vi "Pulsed BPSK Modem.vi"() -> ()   [LabVIEW 2025]
uses:
  Shared/Pulse BPSK Configuration.ctl
  chdr/CHDR Header Layout.ctl
  <vilib>/Platform/TimedLoop/XDataNode/timing_clust.ctl
  <vilib>/Platform/TimedLoop/XDataNode/nitl_modes.ctl
  <vilib>/Platform/TimedLoop/XDataNode/wakeup.ctl
  <vilib>/DLsc/v1/FPGA/DLsc/Endpoint/Data Transfer Type.ctl
  <vilib>/DLsc/v1/FPGA/Aurora 64b66b/Aurora Port Identifier.ctl
  Shared/Public/Demodulator Control.ctl
  <vilib>/rvi/Emulation/niFpgaSctlEmulationGetInTimedLoop.vi
  <vilib>/rvi/Emulation/niFpgaEmulationReportErrorSimple.vi
  <vilib>/rvi/Emulation/niFpgaGetClockAttributes.vi
  <vilib>/rvi/Emulation/niFpgaCriticalErrorInLSC.vi
  <vilib>/eio/utilities/niEioResolveVilibRelativePath.vi
  <vilib>/rvi/interface/RandomDataEmulation/niFpgaRandomDataHandleErrors.vi
  <instrlib>/_niInstr/Basic Elements/v1/FPGA/Private/Count Up U32.vi
  <vilib>/rvi/Memory/Memory_Emulation/nirvimemoryFastEmulation.vi
  <vilib>/rvi/Memory/Memory_Emulation/nirvimemoryEmulation.vi
  <vilib>/rvi/Emulation/niFpgaEmulationIsFPGAContextNoSignature.vi
  <vilib>/rvi/DataTransferAndStorage/Container/Common/niFpgaContainerGetUniqueNameForEmu.vi
  <vilib>/rvi/Emulation/niFpgaProcessEmulError.vi
  <vilib>/rvi/errors/nirviReportUnexpectedCaseInternalError (U32).vi
  <vilib>/rvi/errors/niFpgaSetErrorForExecOnDevCompSimple.vi
  <vilib>/rvi/eio/common/nirviEmuReportErrorAndStop.vi
  <vilib>/rvi/FIFO/Fifo_Resource/nirvififoEmulationSetSize.vi
  <vilib>/rvi/FIFO/Fifo_Resource/nirviFifoEmulationQueueMgr.vi
  <instcachedir>/0/nirviFifoEmulationQueueMgr_E5CAEC123FF24DC58D834DCA3CDAA9B5.lvgen/nirviFifoEmulationQueueMgr_E5CAEC123FF24DC58D834DCA3CDAA9B5_015.vi
  <vilib>/Utility/error.llb/Clear Errors.vi
  <vilib>/rvi/FIFO/Fifo_Resource/nirvififoEmulationCreateLock.vi
  <vilib>/rvi/FIFO/Fifo_Resource/nirvififoEmulationObtainLock.vi
  <vilib>/rvi/FIFO/Fifo_Resource/nirvififoEmulationReleaseLock.vi
  <vilib>/rvi/occurrence/nirviWaitOnOccurrenceBase.vi
  <vilib>/rvi/errors/nirviReportUnexpectedCaseInternalError.vi
  <vilib>/rvi/DataTransferAndStorage/Container/Common/niFpgaContainerSetEmuInfo.vi
  <vilib>/DLsc/v1/FPGA/Aurora 64b66b/Create DX Advanced.vi
  <vilib>/DLsc/v1/FPGA/DLsc/Endpoint/Read Data Stream with Framing 256 Bits.vi
  <instrlib>/_niInstr/Data Formatting/v1/FPGA/Private/Convert/Boolean Array to U32 Array.vi
  <instrlib>/_niInstr/Basic Elements/v1/FPGA/Private/Count Up U64.vi
  <instrlib>/_niInstr/Data Formatting/v1/FPGA/Private/Convert/U32 array to Boolean Array.vi
  <vilib>/DLsc/v1/FPGA/DLsc/Endpoint/Write Data Stream with Framing 256 Bits.vi
  <vilib>/rvi/interface/RandomDataEmulation/nirviRandomDataMultiElementFPGAFIFO.vi
  <instcachedir>/0/nirviRandomDataMultiElementFPGAFIFO_BE2FF10D3D6E420AB0291A02835C249E.lvgen/nirviRandomDataMultiElementFPGAFIFO_BE2FF10D3D6E420AB0291A02835C249E_001.vi
  <instcachedir>/0/nirviRandomDataMultiElementFPGAFIFO_BE2FF10D3D6E420AB0291A02835C249E.lvgen/nirviRandomDataMultiElementFPGAFIFO_BE2FF10D3D6E420AB0291A02835C249E_005.vi
  <vilib>/rvi/FIFO/Fifo_Resource/nirvififoEmulationDetermineInputValidOut.vi
  <vilib>/Platform/TimedLoop/XDataNode/XDataNode.xnode
  <vilib>/rvi/DataTransferAndStorage/Container/XNode/niFpgaContainer.xnode
  <vilib>/rvi/interface/RandomDataEmulation/nirviRandomDataFpgaReadWriteTemplate.vi
  <vilib>/rvi/FIFO/Fifo_Resource/nirvififoEmulationRead.vi
  <vilib>/rvi/LocalResourceManager/LocalResourceManager.xnode
  <vilib>/rvi/interface/RandomDataEmulation/nirviRandomDataFpgaMultiElementTemplate.vi
  <vilib>/rvi/FIFO/Fifo_Resource/nirvififoEmulationWrite.vi
  Shared/BER/FPGA/BER/BER.lvclass
  <vilib>/Platform/TimedLoop/XDataNode/XDNodeRunTimeDep.lvlib
  <instrlib>/_niInstr/FIFO Register Bus/v1/FPGA/niInstr FIFO Register Bus v1 FPGA.lvclass
  <instrlib>/_niInstr/Basic Elements/v1/FPGA/niInstr Basic Elements v1 FPGA.lvlib
  Shared/Pulsed BPSK Modem Shared.lvlib
  Shared/Modems Shared.lvlib
  Shared/AWGN/FPGA/AWGN FPGA.lvlib
  Shared/FIR/FIR.lvlib
  <vilib>/DLsc/v1/FPGA/DLsc/Endpoint/Endpoint.lvclass
  <vilib>/DLsc/v1/FPGA/DLsc/Collection/Endpoint Collection.lvclass
  Shared/AGC/AGC v1 FPGA.lvlib
  <vilib>/DLsc/v1/FPGA/Aurora 64b66b/DLsc Aurora 64b66b v1 FPGA.lvlib
  chdr/CHDR Support.lvlib
  <instrlib>/_niInstr/Data Formatting/v1/FPGA/niInstr Data Formatting v1 FPGA.lvlib
panel:
  out "header count.1":u64
  out "error detection.1":T1
  out "last_timestamp.1":u64
  out "last_header.1":T2
  out "header count.0":u64
  out "error detection.0":T1
  out "last_timestamp.0":u64
  out "last_header.0":T2
  out "bit stream length.1":u32
  in  "update bit generation.1":bool
  in  "preamble write.1":cluster{"address":u32, "write":bool, "value":u8}
  out "current threshold.1":fxp<+/-,15,15>
  in  "preamble.1":i32=449838109 format="%.0x"
  in  "frequency tracking k1.1":fxp<+/-,25,-2>
  in  "frequency tracking k2.1":fxp<+/-,20,-6>
  out "demodulated bits overflow.1":bool
  out "constellation IQ overflow.1":bool
  in  "aurora debug.1":bool
  in  "demodulator control.1":i16
  in  "frame length.1":u16
  out "demodulated bits to BER overflow.1":bool
  in  "threshold precentile.1":fxp<+/-,10,1>=0.80078125 format="%#_10g"
  in  "match filter coefficients.1":T3
  out "aurora.1":bool
  out "current level.1":fxp<+,32,3>
  in  "AGC configurations.1":T4={"k1"=0.0, "k2"=0.0, "target level"=0.0, "level threshold"=0.20001220703125} {"level threshold" format="%#_16g"}
  out "AGC gain.1":fxp<+,19,3>
  in  "reset demodulator.1":bool
  out "pulse buffer underflow.1":bool
  in  "pulse configuration.1":T5={"On Symbol Count"=0, "Off Symbol Count"=7, "filter length"=15, "Preamble Count"=0}
  out "modulated data overflow.1":bool
  out "sink overflow.1":bool
  in  "clear debug.1":bool
  out "pulse control overflow.1":bool
  in  "reset modulator.1":bool
  in  "pulse shaping filter coefficients odd.1":T3
  in  "pulse shaping filter coefficients even.1":T3
  in  "enable modulator.1":bool
  in  "modulator configurations.1":T6 {"power scaling" format="%.16g"; "AWGN scaling" format="%.16g"}
  out "output fifo elements.1":u32
  in  "aurora frame length.1":u16
  in  "header parameters.1":T7
  in  "header parameters.0":T7
  in  "aurora frame length.0":u16
  out "output fifo elements.0":u32
  in  "reset demodulator.0":bool
  out "AGC gain.0":fxp<+,19,3>
  in  "AGC configurations.0":T4={"k1"=0.0, "k2"=0.0, "target level"=0.0, "level threshold"=0.20001220703125} {"level threshold" format="%#_16g"}
  in  "modulator configurations.0":T6 {"power scaling" format="%.16g"; "AWGN scaling" format="%.16g"}
  out "current level.0":fxp<+,32,3>
  out "aurora.0":bool
  in  "match filter coefficients.0":T3
  in  "threshold precentile.0":fxp<+/-,10,1>=0.80078125 format="%#_10g"
  in  "enable modulator.0":bool
  in  "pulse shaping filter coefficients even.0":T3
  in  "pulse shaping filter coefficients odd.0":T3
  out "demodulated bits to BER overflow.0":bool
  in  "preamble write.0":cluster{"address":u32, "write":bool, "value":u8}
  out "bit stream length.0":u32
  in  "update bit generation.0":bool
  in  "reset modulator.0":bool
  out "pulse buffer underflow.0":bool
  in  "pulse configuration.0":T5={"On Symbol Count"=0, "Off Symbol Count"=7, "filter length"=15, "Preamble Count"=0}
  out "modulated data overflow.0":bool
  out "sink overflow.0":bool
  in  "clear debug.0":bool
  out "pulse control overflow.0":bool
  in  "frame length.0":u16
  in  "demodulator control.0":i16
  in  "aurora debug.0":bool
  out "constellation IQ overflow.0":bool
  out "demodulated bits overflow.0":bool
  in  "frequency tracking k2.0":fxp<+/-,20,-6>
  in  "frequency tracking k1.0":fxp<+/-,25,-2>
  in  "preamble.0":i32=449838109 format="%.0x"
  out "current threshold.0":fxp<+/-,15,15>
  in  "fifo reg bus ctrl 0":u32
  out "fifo reg bus data 0":u64
  out "fifo reg bus status 0":u32
  # "Port 8 - Modulator/Demodulator"
  # "Port 9 - Modulator/Demodulator"
  # "Instruction Framework Host Interface. Please do not modify"
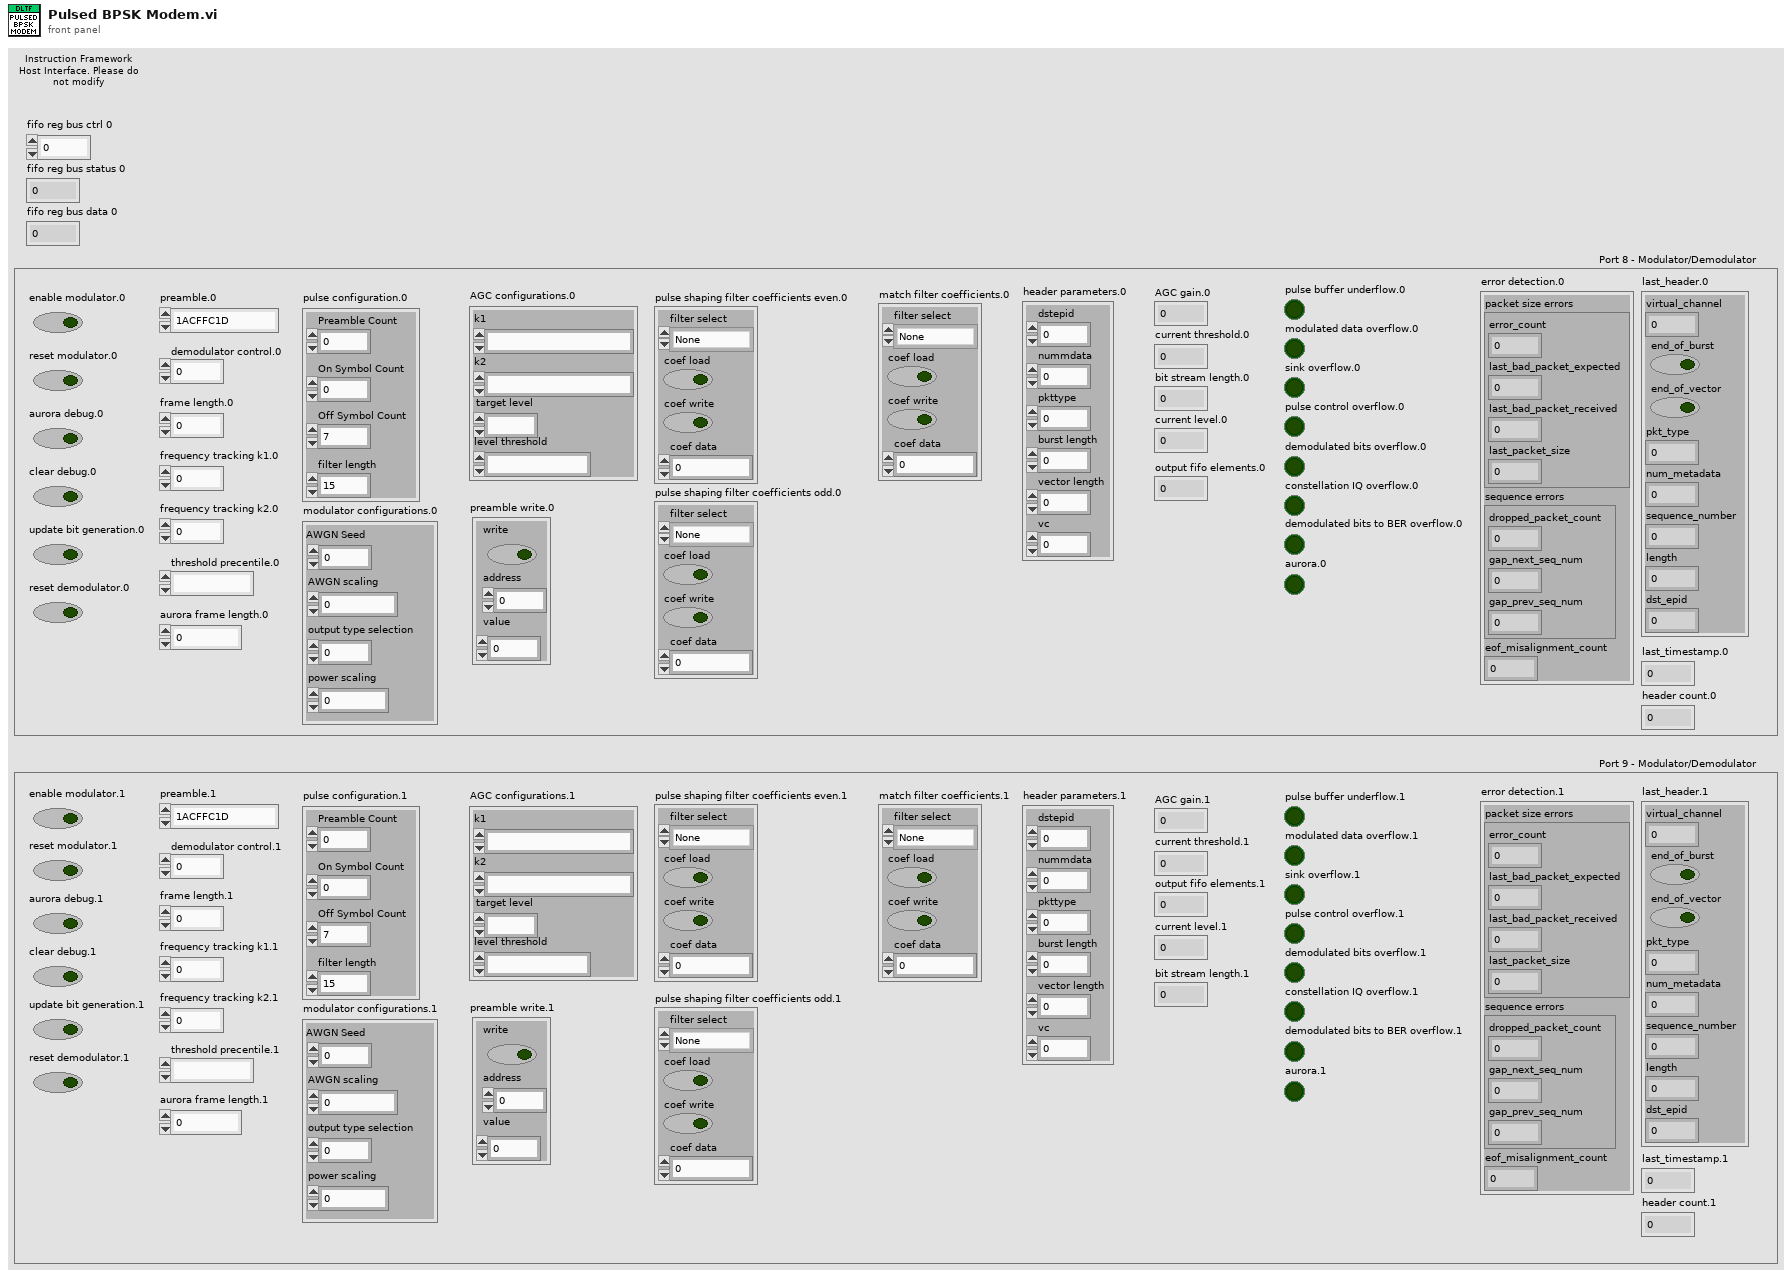
[diagram p1: front panel]
types:
  T1 = cluster{"packet size errors":cluster{"error_count":u64, "last_bad_packet_expected":u16, "last_bad_packet_received":u16, "last_packet_size":u16}, "sequence errors":cluster{"dropped_packet_count":u64, "gap_next_seq_num":u16, "gap_prev_seq_num":u16}, "eof_misalignment_count":u64}
  T2 = typedef "CHDR Support.lvlib/CHDR Header Layout.ctl" = cluster{"virtual_channel":fxp<+,6,6>, "end_of_burst":bool, "end_of_vector":bool, "pkt_type":fxp<+,3,3>, "num_metadata":fxp<+,5,5>, "sequence_number":u16, "length":u16, "dst_epid":u16}
  T3 = cluster{"filter select":enum8{"None", "I Inline", "I Cross", "Q Cross", "Q Inline"}, "coef load":bool, "coef write":bool, "coef data":fxp<+/-,18,1>}
  T4 = cluster{"k1":fxp<+,17,-4>, "k2":fxp<+,17,-8>, "target level":fxp<+,18,2>, "level threshold":fxp<+,18,4>}
  T5 = typedef "Modems Shared.lvlib/Pulse BPSK Configuration.ctl" = cluster{"On Symbol Count":u16, "Off Symbol Count":u16, "filter length":u16, "Preamble Count":u16}
  T6 = cluster{"AWGN Seed":fxp<+,25,25>, "AWGN scaling":fxp<+,16,0>, "output type selection":i16, "power scaling":fxp<+,16,0>}
  T7 = cluster{"dstepid":u16, "nummdata":fxp<+,5,5>, "pkttype":fxp<+,3,3>, "burst length":u16, "vector length":u16, "vc":fxp<+,6,6>}
  T8 = typedef "DLsc v1 FPGA.lvlib/Endpoint.lvclass/Data Transfer Type.ctl" = enum16{"u32 1spc", "u32 2spc", "u32 4spc", "u32 8spc", "u32 16spc", "u32 32spc"}
  T9 = typedef "DLsc Aurora 64b66b v1 FPGA.lvlib/Aurora Port Identifier.ctl" = enum16{"Port 0", "Port 1", "Port 2", "Port 3", "Port 4", "Port 5", "Port 6", "Port 7", "Port 8", "Port 9", "Port 10", "Port 11", "Ports 0-1", "Ports 2-3", "Ports 4-5", "Ports 6-7", "Ports 8-9", "Ports 10-11", "Ports 0-3", "Ports 4-7", "Ports 8-11"}
  T10 = typedef "XDNodeRunTimeDep.lvlib/timing_clust.ctl" = cluster{"Expected End [f-1]":u64, "Actual End [f-1]":u64, "Finished Late? [f-1]":bool, "Expected End [i-1]":u64, "Actual End [i-1]":u64, "Finished Late? [i-1]":bool, "Expected Start [i]":u64, "Actual Start [i]":u64, "Expected Start [f]":u64, "Actual Start [f]":u64, "Source Name":string, "Structure Name":string, "Period":i64, "Deadline":i64, "Offset":i64, "Start":i64, "Priority":i32, "Timeout":i32, "Mode":T11, "Wakeup Reason":T12, "Error":errorcluster, "Source Type":string, "Secondary Source Type":string, "Global End Time":u64, "Global Start Time":u64, "Frame Duration":u64, "Iteration Duration":u64, "Assigned CPU":i32, "I/O Scan Engine Mode":u32}
  T11 = typedef "XDNodeRunTimeDep.lvlib/nitl_modes.ctl" = enum32{"No Change", "Process missed periods, maintain original phase", "Discard missed periods, maintain original phase", "Process missed periods, ignore original phase", "Discard missed periods, ignore original phase"}
  T12 = typedef "XDNodeRunTimeDep.lvlib/wakeup.ctl" = enum32{"Normal", "Aborted", "Asynchronous wakeup", "Timing source error", "Timed loop error", "Timeout"}
  T13 = typedef "Pulsed BPSK Modem Shared.lvlib/Demodulator Control.ctl" = i16
  T14 = cluster{"dropped_packet_count":u64, "gap_next_seq_num":u16, "gap_prev_seq_num":u16}
  T15 = cluster{"error_count":u64, "last_bad_packet_expected":u16, "last_bad_packet_received":u16, "last_packet_size":u16}
  T16 = cluster{"magnitude":fxp<+,16,2>, "phase":fxp<+/-,16,1>, "output valid":bool}[]
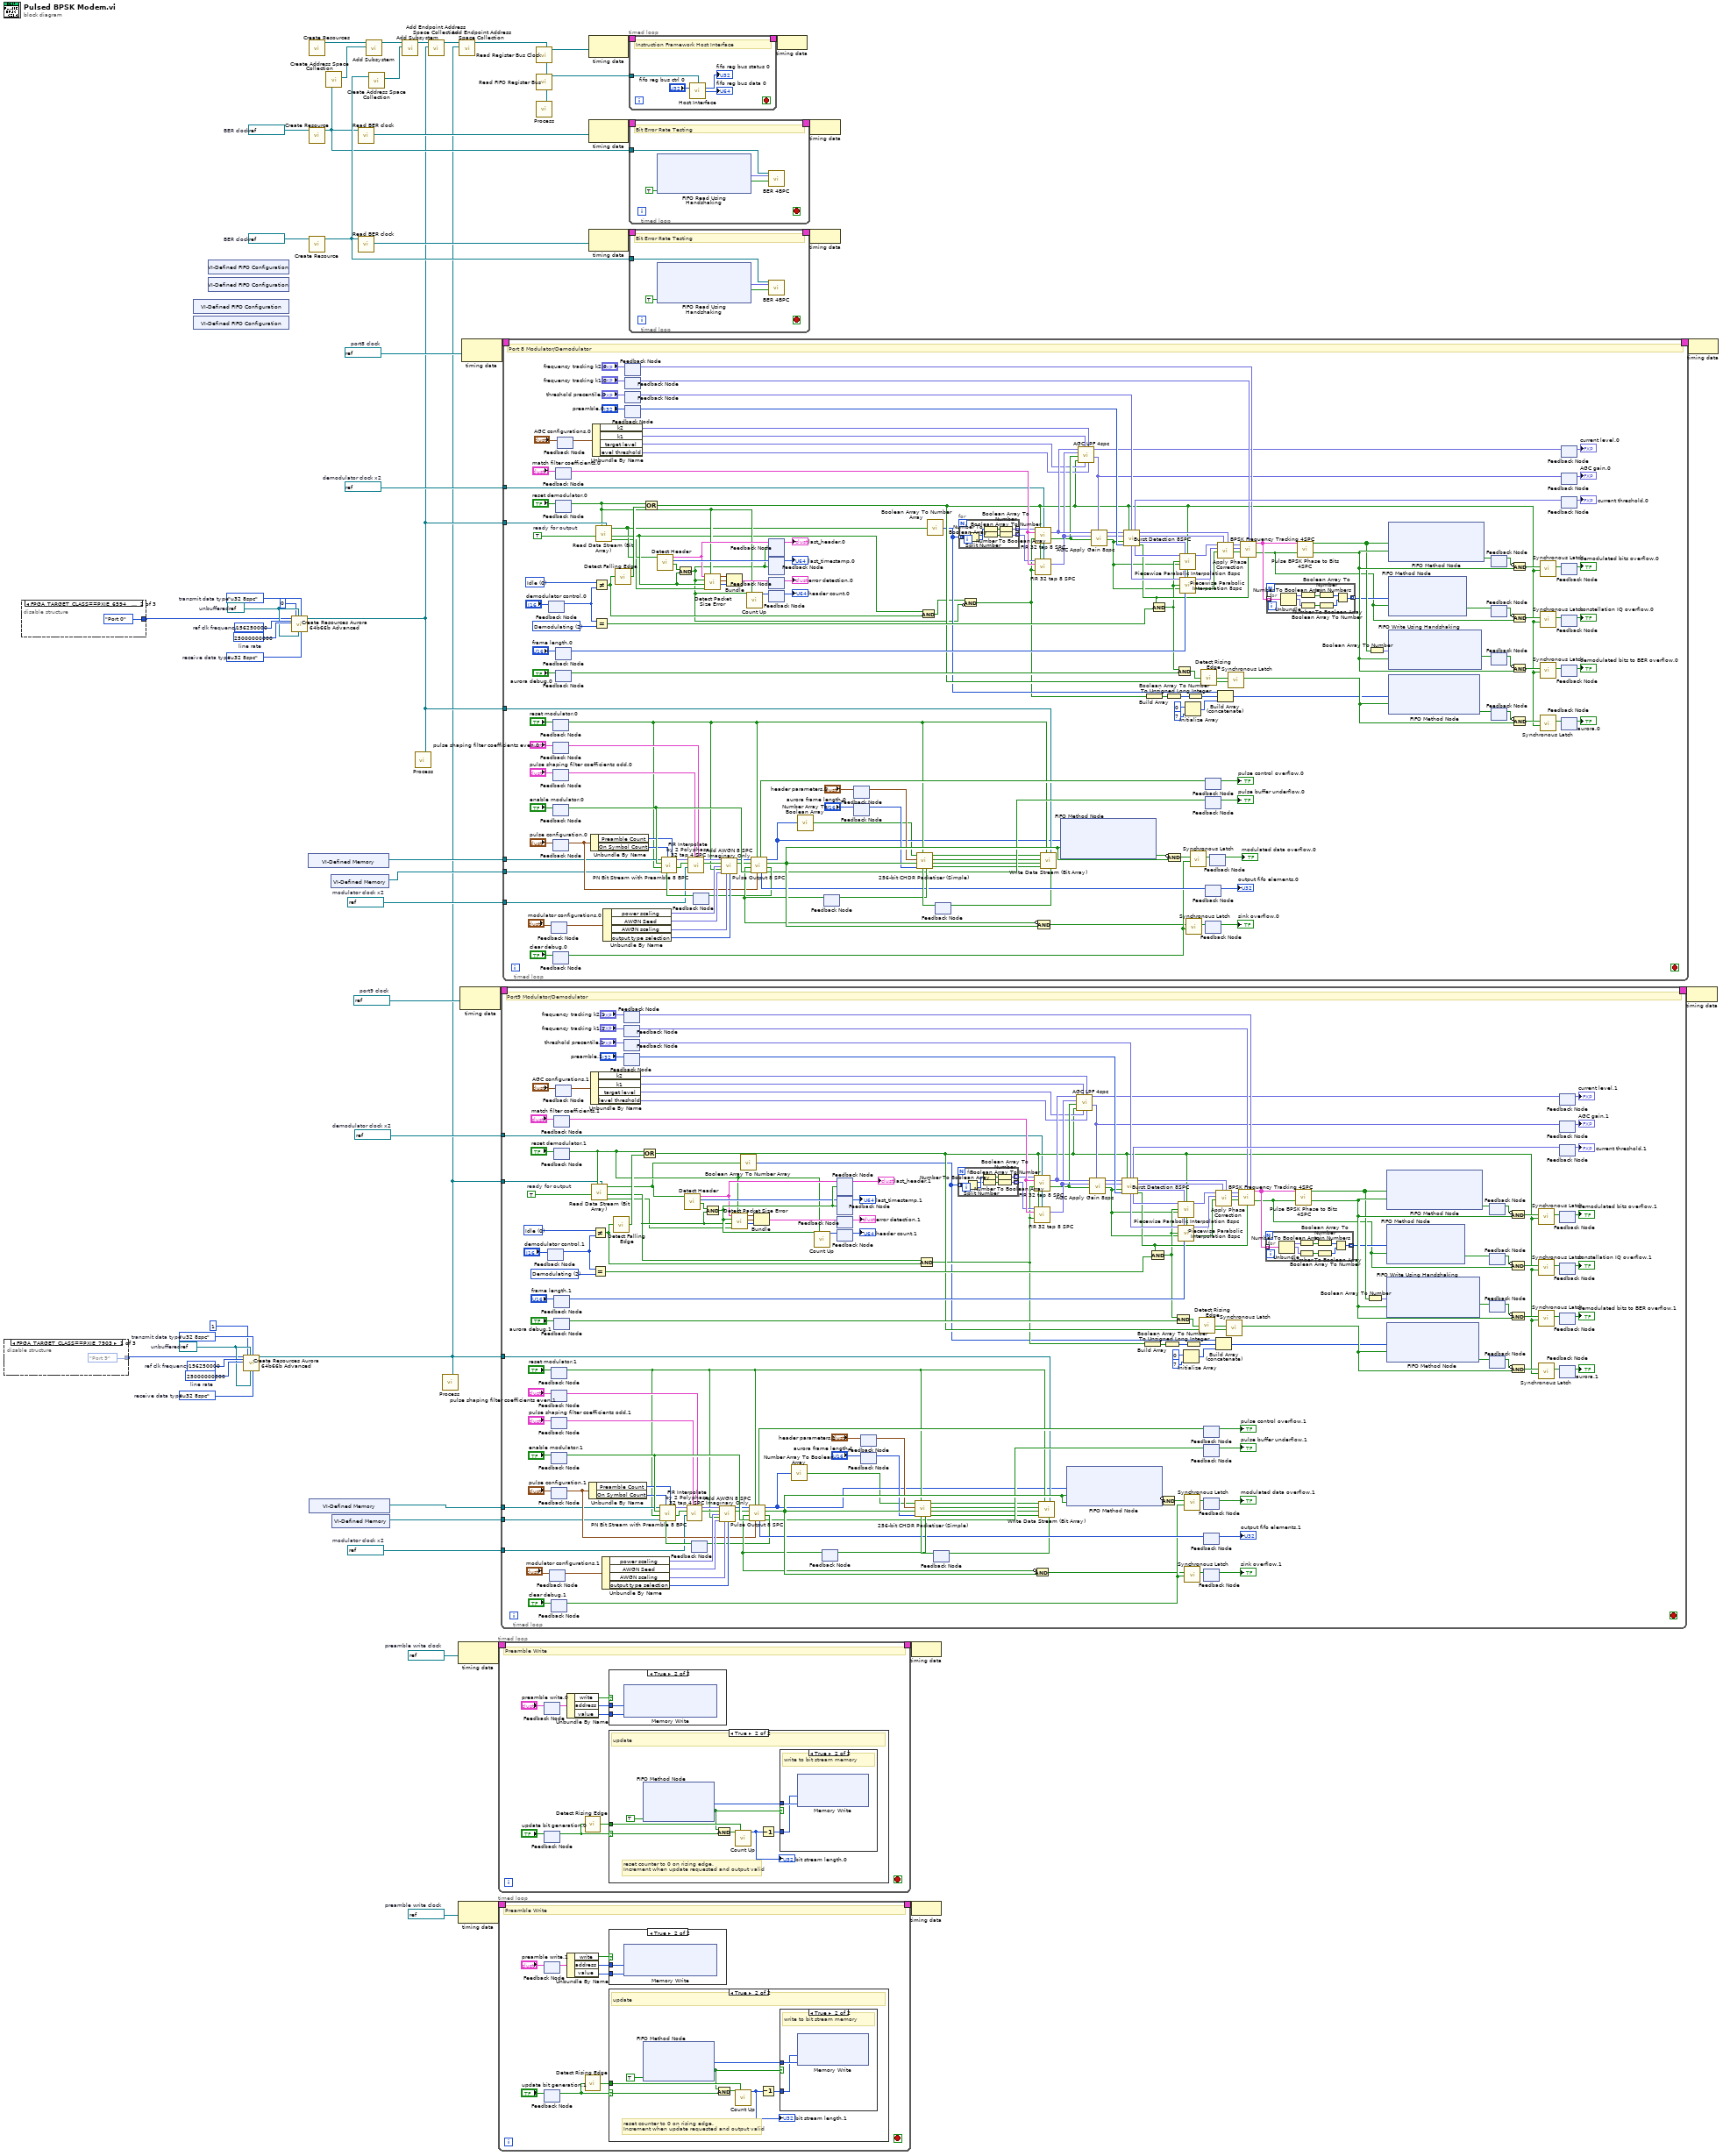
[diagram p0: block diagram]
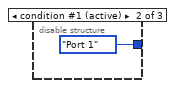
[diagram p2: hidden frame]
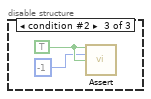
[diagram p3: hidden frame]
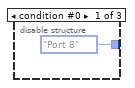
[diagram p4: hidden frame]
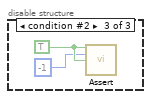
[diagram p5: hidden frame]
diagram:
  w4 = refnum<k21> refnum  # unbuffered
  w5 = Data_Transfer_Type."u32 8spc"  # transmit data type
  w7 = u64 25000000000  # line rate
  w6 = u64 156250000  # ref clk frequency
  w8 = Data_Transfer_Type."u32 8spc"  # receive data type
  w10 = refnum<k21> refnum  # unbuffered
  w11 = Data_Transfer_Type."u32 8spc"  # transmit data type
  w13 = u64 25000000000  # line rate
  w12 = u64 156250000  # ref clk frequency
  w14 = Data_Transfer_Type."u32 8spc"  # receive data type
  w26 = refnum<k21> "120MHz"  # BER clock
  w29 = refnum<k21> "120MHz"  # preamble write clock
  w32 = refnum<k21> "240MHz"  # modulator clock x2
  w33 = refnum<k21> "240MHz"  # demodulator clock x2
  w42 = refnum<k21> "240MHz"  # demodulator clock x2
  w43 = refnum<k21> "120MHz"  # port8 clock
  w37 = refnum<k21> "240MHz"  # modulator clock x2
  w47 = refnum<k21> "120MHz"  # BER clock
  w34 = refnum<k21> "120MHz"  # port9 clock
  w51 = refnum<k21> "120MHz"  # preamble write clock
  n1 = disable-structure shown="FPGA_TARGET_CLASS==PXIE_7903" {
    disable-tunnel: [Aurora_Port_Identifier."Port 9" ("aurora port identifier") Aurora_Port_Identifier."Port 1" ("aurora port identifier") _] -> w1
    frame condition #0 {
    }
    frame condition #1 (active) {
    }
    frame condition #2 {
      w61 = TRUE ("assert")
      n2 = call <instrlib>:"Assert.vi"("assert"=w61, "error code"=-1, "enable show error"=w61) -> ()  [unwired: 13 in]
    }
  }
  n3 = disable-structure shown="FPGA_TARGET_CLASS==PXIE_6594__KU15P_" {
    disable-tunnel: [Aurora_Port_Identifier."Port 8" ("aurora port identifier") Aurora_Port_Identifier."Port 0" ("aurora port identifier") _] -> w2
    frame condition #0 {
    }
    frame condition #1 (active) {
    }
    frame condition #2 {
      w65 = TRUE ("assert")
      n4 = call <instrlib>:"Assert.vi"("assert"=w65, "error code"=-1, "enable show error"=w65) -> ()  [unwired: 13 in]
    }
  }
  n5 = xnode "VI-Defined FIFO Configuration"() -> ()  [unwired: 1 out]
  n6 = xnode "VI-Defined FIFO Configuration"() -> ()  [unwired: 1 out]
  n7 = xnode "VI-Defined FIFO Configuration"() -> ()  [unwired: 1 out]
  n8 = xnode "VI-Defined FIFO Configuration"() -> ()  [unwired: 1 out]
  n9 = call-poly <vilib>:"Create Resources Aurora 64b66b Advanced.vi"("aurora port identifier"=w1, "ref clk frequency"=w12, "line rate"=w13, "instance (0)"=u8 1, "transmit buffer process clock"=w10, "receive buffer process clock"=w10, "transmit data type"=w11, "receive data type"=w14) -> ("endpoint"=w15:refnum<class "Endpoint.lvclass">)  [unwired: 11 in]
  n10 = call-poly <vilib>:"Create Resources Aurora 64b66b Advanced.vi"("aurora port identifier"=w2, "ref clk frequency"=w6, "line rate"=w7, "instance (0)"=u8 0, "transmit buffer process clock"=w4, "receive buffer process clock"=w4, "transmit data type"=w5, "receive data type"=w8) -> ("endpoint"=w16:refnum<class "Endpoint.lvclass">)  [unwired: 11 in]
  n11 = xnode "VI-Defined Memory"() -> ("Memory Out"=w39:refnum<k21>)
  n12 = call <vilib>:"Create Resources.vi"() -> ("endpoint collection"=w44:refnum<class "Endpoint Collection.lvclass">)  [unwired: 11 in]
  n13 = call "Create Resource.vi"("BER clock"=w26) -> ("BER"=w17:refnum<class "BER.lvclass">)  [unwired: 10 in]
  n14 = call "Create Resource.vi"("BER clock"=w47) -> ("BER"=w22:refnum<class "BER.lvclass">)  [unwired: 10 in]
  n15 = xnode "VI-Defined Memory"() -> ("Memory Out"=w28:refnum<k21>)
  n16 = call-dynamic "Create Address Space Collection.vi"("BER"=w17) -> ("address space collection"=w21:refnum<class "Address Space Collection.lvclass">)  [unwired: 9 in, 1 out]
  n17 = xnode "VI-Defined Memory"() -> ("Memory Out"=w38:refnum<k21>)
  n18 = xnode "VI-Defined Memory"() -> ("Memory Out"=w27:refnum<k21>)
  n19 = call "Read BER clock.vi"("BER"=w17) -> ("BER clock"=w23:refnum<k21>)  [unwired: 10 in]
  n20 = call "Read BER clock.vi"("BER"=w22) -> ("BER clock"=w48:refnum<k21>)  [unwired: 10 in]
  n21 = call <vilib>:"Add Subsystem.vi"("subsystems"=w21, "endpoint collection in"=w44) -> ("endpoint collection out"=w20:refnum<class "Endpoint Collection.lvclass">)  [unwired: 9 in]
  n22 = call-dynamic "Create Address Space Collection.vi"("BER"=w22) -> ("address space collection"=w18:refnum<class "Address Space Collection.lvclass">)  [unwired: 9 in, 1 out]
  n23 = call <vilib>:"Add Subsystem.vi"("subsystems"=w18, "endpoint collection in"=w20) -> ("endpoint collection out"=w19:refnum<class "Endpoint Collection.lvclass">)  [unwired: 9 in]
  n24 = call <vilib>:"Process.vi"("endpoint"=w16) -> ()  [unwired: 11 in]
  n25 = call <vilib>:"Add Endpoint Address Space Collection.vi"("endpoint"=w16, "endpoint collection in"=w19) -> ("endpoint collection out"=w41:refnum<class "Endpoint Collection.lvclass">)  [unwired: 9 in]
  n26 = call <vilib>:"Process.vi"("endpoint"=w15) -> ()  [unwired: 11 in]
  n27 = node-c288(w51) -> (w53:T10)
  n28 = node-c288(w29) -> (w31:T10)
  n29 = call <vilib>:"Add Endpoint Address Space Collection.vi"("endpoint"=w15, "endpoint collection in"=w41) -> ("endpoint collection out"=w40:refnum<class "Endpoint Collection.lvclass">)  [unwired: 9 in]
  n30 = node-c288(w34) -> (w36:T10)
  n31 = node-c288(w43) -> (w55:T10)
  n32 = timed-loop {
    timing: w53 -> [_]
    timing-out: [_] -> w52
    stop <- _ stop-if-true
    # "Preamble Write"
    n33 = feedback #1() -> (w66:cluster{"address":u32, "write":bool, "value":u8})  [unwired: 1 in]
    n34 = feedback-in #1("preamble write.0") -> ()
    n35 = feedback #2() -> (w72:bool)  [unwired: 1 in]
    n36 = feedback-in #2("update bit generation.0") -> ()
    n37 = Unbundle By Name(w66) -> ("write"=w69:bool, "address"=w70:u32, "value"=w68:u8)
    n38 = call <instrlib>:"Detect Rising Edge.vi"("signal"=w72) -> ("edge detected"=w71:bool)  [unwired: 14 in]
    n39 = case shown="True" w69 {
      tunnel: w70 -> [_ w75]
      tunnel: w68 -> [_ w74]
      frame False {
      }
      frame True {
        n40 = xnode ("Memory Write")("Address"=w75, "Data"=w74) -> ()  [unwired: 1 in, 1 out]
      }
    }
    n41 = case shown="True" w72 {
      selector: w72 -> [_ w80]
      tunnel: w71 -> [_ w83]
      frame False {
        # "Don't update"
      }
      frame True {
        # "reset counter to 0 on rising edge.\nIncrement when update requested and output valid"
        # "update"
        n42 = xnode ("FIFO Method Node")("Ready for Output"=TRUE) -> ("Element"=w82:u8, "Output Valid"=w78:bool)  [unwired: 1 in, 1 out]
        n43 = Compound Arithmetic op=AND(w78, w80) -> (w79:bool)
        n44 = call-poly <instrlib>:"Count Up.vi"("increment"=w79, "reset"=w83) -> ("count out"=w76:u32)  [unwired: 13 in]
        "bit stream length.0" <- w76
        n45 = Decrement(x=w76) -> (x-1=w77:u32)
        n46 = case shown="True" w78 {
          tunnel: w77 -> [_ w84]
          tunnel: w82 -> [_ w85]
          frame False {
            # "nothing to write"
          }
          frame True {
            # "write to bit stream memory"
            n47 = xnode ("Memory Write")("Address"=w84, "Data"=w85) -> ()  [unwired: 1 in, 1 out]
          }
        }
      }
    }
  }
  n48 = timed-loop {
    timing: w31 -> [_]
    timing-out: [_] -> w30
    stop <- _ stop-if-true
    # "Preamble Write"
    n49 = feedback #3() -> (w88:cluster{"address":u32, "write":bool, "value":u8})  [unwired: 1 in]
    n50 = feedback-in #3("preamble write.1") -> ()
    n51 = feedback #4() -> (w94:bool)  [unwired: 1 in]
    n52 = feedback-in #4("update bit generation.1") -> ()
    n53 = Unbundle By Name(w88) -> ("write"=w91:bool, "address"=w92:u32, "value"=w90:u8)
    n54 = call <instrlib>:"Detect Rising Edge.vi"("signal"=w94) -> ("edge detected"=w93:bool)  [unwired: 14 in]
    n55 = case shown="True" w91 {
      tunnel: w92 -> [_ w97]
      tunnel: w90 -> [_ w96]
      frame False {
      }
      frame True {
        n56 = xnode ("Memory Write")("Address"=w97, "Data"=w96) -> ()  [unwired: 1 in, 1 out]
      }
    }
    n57 = case shown="True" w94 {
      selector: w94 -> [_ w102]
      tunnel: w93 -> [_ w105]
      frame False {
        # "Don't update"
      }
      frame True {
        # "reset counter to 0 on rising edge.\nIncrement when update requested and output valid"
        # "update"
        n58 = xnode ("FIFO Method Node")("Ready for Output"=TRUE) -> ("Element"=w104:u8, "Output Valid"=w100:bool)  [unwired: 1 in, 1 out]
        n59 = Compound Arithmetic op=AND(w100, w102) -> (w101:bool)
        n60 = call-poly <instrlib>:"Count Up.vi"("increment"=w101, "reset"=w105) -> ("count out"=w98:u32)  [unwired: 13 in]
        "bit stream length.1" <- w98
        n61 = Decrement(x=w98) -> (x-1=w99:u32)
        n62 = case shown="True" w100 {
          tunnel: w99 -> [_ w106]
          tunnel: w104 -> [_ w107]
          frame False {
            # "nothing to write"
          }
          frame True {
            # "write to bit stream memory"
            n63 = xnode ("Memory Write")("Address"=w106, "Data"=w107) -> ()  [unwired: 1 in, 1 out]
          }
        }
      }
    }
  }
  n64 = timed-loop {
    timing: w36 -> [_]
    timing-out: [_] -> w35
    tunnel: w33 -> [w191]
    tunnel: w28 -> [w141]
    tunnel: w27 -> [w140]
    tunnel: w32 -> [w139]
    tunnel: w15 -> [w120]
    tunnel: w15 -> [w115]
    stop <- _ stop-if-true
    w138 = TRUE  # ready for output
    w268 = T13 2 items=["Idle", "Initial Threshold Detection", "Demodulating"] ("demodulation control")
    w271 = T13 0 items=["Idle", "Initial Threshold Detection", "Demodulating"] ("demodulation control")
    # "Port9 Modulator/Demodulator"
    n65 = feedback #5() -> (w269:i16)  [unwired: 1 in]
    n66 = feedback-in #5("demodulator control.1") -> ()
    n67 = feedback #6() -> (w175:T6)  [unwired: 1 in]
    n68 = feedback-in #6("modulator configurations.1") -> ()
    n69 = feedback #7() -> (w119:bool)  [unwired: 1 in]
    n70 = feedback-in #7("reset modulator.1") -> ()
    n71 = feedback #8() -> (w167:T3)  [unwired: 1 in]
    n72 = feedback-in #8("pulse shaping filter coefficients even.1") -> ()
    n73 = feedback #9() -> (w166:T3)  [unwired: 1 in]
    n74 = feedback-in #9("pulse shaping filter coefficients odd.1") -> ()
    n75 = feedback #10() -> (w180:bool)  [unwired: 1 in]
    n76 = feedback-in #10("enable modulator.1") -> ()
    n77 = feedback #11() -> (w142:T5)  [unwired: 1 in]
    n78 = feedback-in #11("pulse configuration.1") -> ()
    n79 = feedback #12() -> (w158:bool)  [unwired: 1 in]
    n80 = feedback-in #12("clear debug.1") -> ()
    n81 = feedback #13() -> (w254:T3)  [unwired: 1 in]
    n82 = feedback-in #13("match filter coefficients.1") -> ()
    n83 = feedback #14() -> (w123:bool)  [unwired: 1 in]
    n84 = feedback-in #14("reset demodulator.1") -> ()
    n85 = feedback #15() -> (w238:u16)  [unwired: 1 in]
    n86 = feedback-in #15("frame length.1") -> ()
    n87 = feedback #16() -> (w211:bool)  [unwired: 1 in]
    n88 = feedback-in #16("aurora debug.1") -> ()
    n89 = feedback-in #17("AGC configurations.1") -> ()
    n90 = feedback #17() -> (w200:T4)  [unwired: 1 in]
    n91 = Unbundle By Name(w142) -> ("Preamble Count"=w147:u16, "On Symbol Count"=w155:u16)
    n92 = Unbundle By Name(w200) -> ("k2"=w198:fxp<+,17,-8>, "k1"=w199:fxp<+,17,-4>, "target level"=w197:fxp<+,18,2>, "level threshold"=w196:fxp<+,18,4>)
    n93 = call-poly <vilib>:"Read Data Stream (Bit Array).vi"("endpoint"=w115, "reset"=w123, "ready for output"=w138) -> ("end of frame"=w114:bool, "output valid"=w124:bool, "data"=w122:bool[])  [unwired: 5 in, 1 out]
    n94 = Not Equal?(x=w271, y=w269) -> (x != y?=w262:bool)
    n95 = Equal?(x=w269, y=w268) -> (x = y?=w242:bool)
    n96 = Unbundle By Name(w175) -> ("power scaling"=w176:fxp<+,16,0>, "AWGN Seed"=w177:fxp<+,25,25>, "AWGN scaling"=w178:fxp<+,16,0>, "output type selection"=w179:i16)
    n97 = call <instrlib>:"Detect Falling Edge.vi"("signal"=w262) -> ("edge detected"=w263:bool)  [unwired: 14 in]
    n98 = feedback #18() -> (w244:fxp<+/-,20,-6>)  [unwired: 1 in]
    n99 = feedback-in #18("frequency tracking k2.1") -> ()
    n100 = feedback #19() -> (w245:fxp<+/-,25,-2>)  [unwired: 1 in]
    n101 = feedback-in #19("frequency tracking k1.1") -> ()
    n102 = feedback #20() -> (w247:fxp<+/-,10,1>)  [unwired: 1 in]
    n103 = feedback-in #20("threshold precentile.1") -> ()
    n104 = feedback #21() -> (w248:i32)  [unwired: 1 in]
    n105 = feedback-in #21("preamble.1") -> ()
    n106 = Compound Arithmetic op=OR(w123, w263) -> (w192:bool)
    n107 = call "Detect Header.vi"("input data"=w122) -> ("header detected"=w134:bool, "timestamp"=w136:u64, "chdr_header"=w135:T2)  [unwired: 8 in]
    n108 = feedback #22() -> (w164:bool)  [unwired: 1 in]
    n109 = call "PN Bit Stream with Preamble 8 BPC.vi"("preamble count"=w147, "ready for output"=w164, "on symbol count"=w155, "bit stream memory"=w140, "reset modulator"=w119, "start modulator"=w180, "preamble memory"=w141) -> ("output valid"=w169:bool, "data"=w168:fxp<+/-,16,1>[])  [unwired: 3 in]
    n110 = call "FIR Interpolate by 2 Polyphase 32 tap 4 SPC.vi"("filter coefficients even"=w167, "filter coefficients odd"=w166, "clock x2"=w139, "input valid"=w169, "data"=w168) -> ("output valid"=w171:bool, "data out"=w170:fxp<+/-,16,2>[])  [unwired: 5 in]
    n111 = Compound Arithmetic op=AND(w134, w124) -> (w137:bool)
    n112 = call "Add AWGN 8 SPC Imaginary Only.vi"("imaginary"=w170, "input valid"=w171, "power scaling"=w176, "reset"=w119, "seed"=w177, "scaling factor"=w178, "Output Type Selection"=w179) -> ("output with noise"=w162:u32[], "output valid"=w163:bool)  [unwired: 7 in]
    n113 = call "Detect Packet Size Error.vi"("reset_pse"=w123, "end of frame"=w114, "input valid"=w124, "packet_header"=w137, "chdr_header"=w135) -> ("eof_misalignment_count"=w129:u64, "sequence errors"=w128:T14, "packet size errors"=w127:T15)  [unwired: 4 in]
    n114 = call-poly <instrlib>:"Boolean Array To Number Array.vi"("data in"=w122) -> ("data out"=w121:u32[])  [unwired: 14 in]
    n115 = Bundle("packet size errors"=w127, "sequence errors"=w128, "eof_misalignment_count"=w129) -> (w131:T1)  [unwired: 1 in]
    n116 = call-poly <instrlib>:"Count Up.vi"("increment"=w137, "reset"=w123) -> ("count out"=w130:u64)  [unwired: 13 in]
    n117 = feedback #23() -> (w157:bool)  [unwired: 1 in]
    n118 = call "Pulse Output 8 SPC.vi"("Pulse Configuration"=w142, "reset"=w119, "enable"=w180, "ready for output"=w157, "input valid"=w163, "8 spc imaginary"=w162) -> ("Pulse Buffer Underflow"=w143:bool, "Ready for Input"=w144:bool, "output valid"=w187:bool, "IQ data out"=w113:u32[], "Number of Elements to Read"=w181:u32, "pulse buffer overflow"=w172:bool)
    n119 = feedback-in #22(w144) -> ()
    n120 = call-poly <instrlib>:"Number Array To Boolean Array.vi"("data in"=w113) -> ("data out"=w112:bool[])  [unwired: 14 in]
    n121 = feedback #24() -> (→"last_header.1":T2)  [unwired: 1 in]
    n122 = feedback-in #24(w135, w137) -> ()
    n123 = feedback #25() -> (→"last_timestamp.1":u64)  [unwired: 1 in]
    n124 = feedback-in #25(w136, w137) -> ()
    n125 = feedback #26() -> (→"error detection.1":T1)  [unwired: 1 in]
    n126 = feedback-in #26(w131) -> ()
    n127 = feedback #27() -> (→"header count.1":u64)  [unwired: 1 in]
    n128 = feedback-in #27(w130) -> ()
    n129 = feedback #28() -> (w184:T7)  [unwired: 1 in]
    n130 = feedback-in #28("header parameters.1") -> ()
    n131 = feedback #29() -> (w186:u16)  [unwired: 1 in]
    n132 = feedback-in #29("aurora frame length.1") -> ()
    n133 = Compound Arithmetic op=AND(w124, w262) -> (w190:bool)
    n134 = feedback #30() -> (w189:bool)  [unwired: 1 in]
    n135 = call "256-bit CHDR Packetizer (Simple).vi"("ready for output"=w189, "reset"=w119, "aurora frame length"=w186, "input valid"=w187, "header parameters"=w184, "data"=w112) -> ("tlast"=w110:bool, "output valid"=w116:bool, "tkeep"=w111:bool[], "data out"=w118:bool[], "ready for input"=w188:bool)  [unwired: 1 in]
    n136 = feedback-in #23(w188) -> ()
    n137 = for {
      tunnel: w121 -> [w286] mode=indexing
      tunnel: [w285] -> w253 mode=indexing
      tunnel: [w284] -> w252 mode=indexing
      n138 = Split Number(x=w286) -> (hi(x)=w289:u16, lo(x)=w290:u16)
      n139 = Number To Boolean Array(number=w290) -> (Boolean array=w288:bool[])
      n140 = Number To Boolean Array(number=w289) -> (Boolean array=w287:bool[])
      n141 = Boolean Array To Number(Boolean array=w288) -> (number=w285:fxp<+/-,16,1>)
      n142 = Boolean Array To Number(Boolean array=w287) -> (number=w284:fxp<+/-,16,1>)
    }
    n143 = call "FIR 32 tap 8 SPC.vi"("data in"=w253, "reset"=w192, "clock x2"=w191, "filter coefficients"=w254, "input valid"=w190) -> ("data out 16.1"=w209:fxp<+/-,16,1>[], "output valid"=w207:bool)  [unwired: 8 in, 1 out]
    n144 = call "FIR 32 tap 8 SPC.vi"("data in"=w252, "reset"=w192, "clock x2"=w191, "filter coefficients"=w254, "input valid"=w190) -> ("data out 16.1"=w208:fxp<+/-,16,1>[])  [unwired: 8 in, 2 out]
    n145 = Compound Arithmetic op=AND(invert w157, w187) -> (w153:bool)
    n146 = call-poly <vilib>:"Write Data Stream (Bit Array).vi"("endpoint"=w120, "reset"=w119, "end of frame"=w110, "input valid"=w116, "byte enable"=w111, "data"=w118) -> ("ready for input"=w117:bool)  [unwired: 5 in]
    n147 = feedback-in #30(w117) -> ()
    n148 = xnode ("FIFO Method Node")("Element"=w113, "Input Valid"=w187) -> ("Ready for Input"=w148:bool)  [unwired: 1 in, 1 out]
    n149 = call "AGC LPF 4spc.vi"("level threshold"=w196, "k 2"=w198, "level"=w197, "k 1"=w199, "reset"=w192, "input valid"=w207, "din img"=w208, "din real"=w209) -> ("AGC gain"=w194:fxp<+,19,3>, "current level"=w203:fxp<+,32,3>)  [unwired: 1 in, 1 out]
    n150 = call "AGC Apply Gain 8spc.vi"("AGC gain"=w194, "input valid"=w207, "din img"=w208, "din real"=w209) -> ("output valid"=w204:bool, "dout img"=w205:fxp<+/-,16,1>[], "dout real"=w206:fxp<+/-,16,1>[])  [unwired: 5 in]
    n151 = call "Burst Detection 8SPC.vi"("x real"=w206, "reset"=w192, "threshold precentile"=w247, "x img"=w205, "input valid"=w204, "preamble"=w248) -> ("Current Threshold"=w246:fxp<+/-,15,15>, "phase correction cos"=w237:fxp<+/-,16,2>, "phase correction sin"=w236:fxp<+/-,16,2>, "timing"=w243:fxp<+,13,0>, "img to interpolator"=w228:fxp<+/-,16,1>[], "real to interpolator"=w229:fxp<+/-,16,1>[], "preamble detected"=w226:bool)  [unwired: 2 in, 1 out]
    n152 = Build Array(w190) -> (w213:bool[])
    n153 = Compound Arithmetic op=AND(w226, w242) -> (w212:bool)
    n154 = Compound Arithmetic op=AND(invert w148, w187) -> (w149:bool)
    n155 = Boolean Array To Number(Boolean array=w213) -> (number=w219:u8)
    n156 = Compound Arithmetic op=AND(w212, w211) -> (w210:bool)
    n157 = call "Piecewise Parabolic Interpolation 8spc.vi"("x[n]"=w229, "u[k]"=w243, "reset"=w192, "preamble found"=w212, "input valid"=w204, "frame length"=w238) -> ("y[n]"=w234:fxp<+/-,16,2>[])  [unwired: 8 in, 1 out]
    n158 = call "Piecewise Parabolic Interpolation 8spc.vi"("x[n]"=w228, "u[k]"=w243, "reset"=w192, "preamble found"=w212, "input valid"=w204, "frame length"=w238) -> ("y[n]"=w233:fxp<+/-,16,2>[], "output valid"=w230:bool)  [unwired: 8 in]
    n159 = Initialize Array(u32 0 ("element"), 7 ("dimension size")) -> (w217:u32[])
    n160 = call <instrlib>:"Synchronous Latch.vi"("clear"=w158, "set"=w149) -> ("out"=w150:bool)  [unwired: 9 in]
    n161 = call <instrlib>:"Synchronous Latch.vi"("clear"=w158, "set"=w153) -> ("out"=w152:bool)  [unwired: 9 in]
    n162 = To Unsigned Long Integer(number=w219) -> (unsigned 32bit integer=w218:u32)
    n163 = call <instrlib>:"Detect Rising Edge.vi"("signal"=w210) -> ("edge detected"=w227:bool)  [unwired: 14 in]
    n164 = feedback #31() -> (→"pulse control overflow.1":bool)  [unwired: 1 in]
    n165 = feedback-in #31(w172) -> ()
    n166 = feedback #32() -> (→"pulse buffer underflow.1":bool)  [unwired: 1 in]
    n167 = feedback-in #32(w143) -> ()
    n168 = feedback #33() -> (→"modulated data overflow.1":bool)  [unwired: 1 in]
    n169 = feedback-in #33(w150) -> ()
    n170 = feedback #34() -> (→"output fifo elements.1":u32)  [unwired: 1 in]
    n171 = feedback-in #34(w181) -> ()
    n172 = feedback #35() -> (→"sink overflow.1":bool)  [unwired: 1 in]
    n173 = feedback-in #35(w152) -> ()
    n174 = call "Apply Phase Correction.vi"("phase correction cos"=w237, "phase correction sin"=w236, "input valid"=w230, "input img"=w233, "input real"=w234) -> ("output valid"=w249:bool, "output img"=w250:fxp<+/-,16,2>[], "output real"=w251:fxp<+/-,16,2>[])  [unwired: 4 in]
    n175 = Build Array (concatenate)(w121, w218, w217) -> (w214:u32[])
    n176 = call <instrlib>:"Synchronous Latch.vi"("clear"=w192, "set"=w227) -> ("out"=w220:bool)  [unwired: 9 in]
    n177 = call "BPSK Frequency Tracking 4SPC.vi"("I data in"=w251, "k1"=w245, "k2"=w244, "Q data in"=w250, "input valid"=w249, "reset"=w226) -> ("polar output"=w235:T16, "output valid"=w231:bool)  [unwired: 7 in, 1 out]
    n178 = for {
      tunnel: [w294] -> w232 mode=indexing
      tunnel: w235 -> [w293] mode=indexing
      n179 = Unbundle(w293) -> ("magnitude"=w292:fxp<+,16,2>, "phase"=w291:fxp<+/-,16,1>)  [unwired: 1 out]
      n180 = Number To Boolean Array(number=w292) -> (Boolean array=w298:bool[])
      n181 = Number To Boolean Array(number=w291) -> (Boolean array=w297:bool[])
      n182 = Boolean Array To Number(Boolean array=w298) -> (number=w296:u16)
      n183 = Boolean Array To Number(Boolean array=w297) -> (number=w295:u16)
      n184 = Join Numbers(hi=w296, lo=w295) -> ((hi.lo)=w294:u32)
    }
    n185 = call "Pulse BPSK Phase to Bits 4SPC.vi"("polar output"=w235, "input valid"=w231) -> ("bit"=w239:bool[], "output valid"=w241:bool)  [unwired: 12 in]
    n186 = Boolean Array To Number(Boolean array=w239) -> (number=w240:fxp<+,4,4>)
    n187 = xnode ("FIFO Method Node")("Element"=w239, "Input Valid"=w241) -> ("Ready for Input"=w267:bool)  [unwired: 1 in, 1 out]
    n188 = xnode ("FIFO Method Node")("Element"=w232, "Input Valid"=w231) -> ("Ready for Input"=w265:bool)  [unwired: 1 in, 1 out]
    n189 = xnode ("FIFO Write Using Handshaking")("Element"=w240, "Input Valid"=w241) -> ("Ready for Input"=w257:bool)  [unwired: 1 in, 1 out]
    n190 = xnode ("FIFO Method Node")("Element"=w214, "Input Valid"=w220) -> ("Ready for Input"=w225:bool)  [unwired: 1 in, 1 out]
    n191 = feedback #36() -> (w266:bool)  [unwired: 1 in]
    n192 = feedback-in #36(w267) -> ()
    n193 = feedback #37() -> (w264:bool)  [unwired: 1 in]
    n194 = feedback-in #37(w265) -> ()
    n195 = feedback #38() -> (w258:bool)  [unwired: 1 in]
    n196 = feedback-in #38(w257) -> ()
    n197 = feedback #39() -> (w221:bool)  [unwired: 1 in]
    n198 = feedback-in #39(w225) -> ()
    n199 = Compound Arithmetic op=AND(invert w266, w241) -> (w279:bool)
    n200 = Compound Arithmetic op=AND(invert w264, w231) -> (w276:bool)
    n201 = Compound Arithmetic op=AND(invert w258, w241) -> (w259:bool)
    n202 = Compound Arithmetic op=AND(invert w221, w220) -> (w222:bool)
    n203 = call <instrlib>:"Synchronous Latch.vi"("clear"=w192, "set"=w279) -> ("out"=w278:bool)  [unwired: 9 in]
    n204 = call <instrlib>:"Synchronous Latch.vi"("clear"=w192, "set"=w276) -> ("out"=w275:bool)  [unwired: 9 in]
    n205 = call <instrlib>:"Synchronous Latch.vi"("clear"=w192, "set"=w259) -> ("out"=w260:bool)  [unwired: 9 in]
    n206 = call <instrlib>:"Synchronous Latch.vi"("clear"=w192, "set"=w222) -> ("out"=w223:bool)  [unwired: 9 in]
    n207 = feedback #40() -> (→"current level.1":fxp<+,32,3>)  [unwired: 1 in]
    n208 = feedback-in #40(w203) -> ()
    n209 = feedback #41() -> (→"AGC gain.1":fxp<+,19,3>)  [unwired: 1 in]
    n210 = feedback-in #41(w194) -> ()
    n211 = feedback #42() -> (→"current threshold.1":fxp<+/-,15,15>)  [unwired: 1 in]
    n212 = feedback-in #42(w246) -> ()
    n213 = feedback #43() -> (→"demodulated bits overflow.1":bool)  [unwired: 1 in]
    n214 = feedback-in #43(w278) -> ()
    n215 = feedback #44() -> (→"constellation IQ overflow.1":bool)  [unwired: 1 in]
    n216 = feedback-in #44(w275) -> ()
    n217 = feedback #45() -> (→"demodulated bits to BER overflow.1":bool)  [unwired: 1 in]
    n218 = feedback-in #45(w260) -> ()
    n219 = feedback #46() -> (→"aurora.1":bool)  [unwired: 1 in]
    n220 = feedback-in #46(w223) -> ()
  }
  n221 = timed-loop {
    timing: w55 -> [_]
    timing-out: [_] -> w54
    tunnel: w42 -> [w384]
    tunnel: w39 -> [w335]
    tunnel: w38 -> [w334]
    tunnel: w37 -> [w333]
    tunnel: w16 -> [w315]
    tunnel: w16 -> [w331]
    stop <- _ stop-if-true
    w332 = TRUE  # ready for output
    w460 = T13 2 items=["Idle", "Initial Threshold Detection", "Demodulating"] ("demodulation control")
    w463 = T13 0 items=["Idle", "Initial Threshold Detection", "Demodulating"] ("demodulation control")
    # "Port 8 Modulator/Demodulator"
    n222 = feedback #47() -> (w461:i16)  [unwired: 1 in]
    n223 = feedback-in #47("demodulator control.0") -> ()
    n224 = feedback #48() -> (w369:T6)  [unwired: 1 in]
    n225 = feedback-in #48("modulator configurations.0") -> ()
    n226 = feedback #49() -> (w311:bool)  [unwired: 1 in]
    n227 = feedback-in #49("reset modulator.0") -> ()
    n228 = feedback #50() -> (w361:T3)  [unwired: 1 in]
    n229 = feedback-in #50("pulse shaping filter coefficients even.0") -> ()
    n230 = feedback #51() -> (w360:T3)  [unwired: 1 in]
    n231 = feedback-in #51("pulse shaping filter coefficients odd.0") -> ()
    n232 = feedback #52() -> (w374:bool)  [unwired: 1 in]
    n233 = feedback-in #52("enable modulator.0") -> ()
    n234 = feedback #53() -> (w336:T5)  [unwired: 1 in]
    n235 = feedback-in #53("pulse configuration.0") -> ()
    n236 = feedback #54() -> (w352:bool)  [unwired: 1 in]
    n237 = feedback-in #54("clear debug.0") -> ()
    n238 = feedback #55() -> (w447:T3)  [unwired: 1 in]
    n239 = feedback-in #55("match filter coefficients.0") -> ()
    n240 = feedback #56() -> (w318:bool)  [unwired: 1 in]
    n241 = feedback-in #56("reset demodulator.0") -> ()
    n242 = feedback #57() -> (w431:u16)  [unwired: 1 in]
    n243 = feedback-in #57("frame length.0") -> ()
    n244 = feedback #58() -> (w404:bool)  [unwired: 1 in]
    n245 = feedback-in #58("aurora debug.0") -> ()
    n246 = feedback-in #59("AGC configurations.0") -> ()
    n247 = feedback #59() -> (w393:T4)  [unwired: 1 in]
    n248 = Unbundle By Name(w336) -> ("Preamble Count"=w341:u16, "On Symbol Count"=w349:u16)
    n249 = Unbundle By Name(w393) -> ("k2"=w391:fxp<+,17,-8>, "k1"=w392:fxp<+,17,-4>, "target level"=w390:fxp<+,18,2>, "level threshold"=w389:fxp<+,18,4>)
    n250 = Not Equal?(x=w463, y=w461) -> (x != y?=w304:bool)
    n251 = Equal?(x=w461, y=w460) -> (x = y?=w435:bool)
    n252 = call-poly <vilib>:"Read Data Stream (Bit Array).vi"("endpoint"=w331, "reset"=w318, "ready for output"=w332) -> ("end of frame"=w309:bool, "output valid"=w317:bool, "data"=w310:bool[])  [unwired: 5 in, 1 out]
    n253 = Unbundle By Name(w369) -> ("power scaling"=w370:fxp<+,16,0>, "AWGN Seed"=w371:fxp<+,25,25>, "AWGN scaling"=w372:fxp<+,16,0>, "output type selection"=w373:i16)
    n254 = call <instrlib>:"Detect Falling Edge.vi"("signal"=w304) -> ("edge detected"=w455:bool)  [unwired: 14 in]
    n255 = feedback #60() -> (w437:fxp<+/-,20,-6>)  [unwired: 1 in]
    n256 = feedback-in #60("frequency tracking k2.0") -> ()
    n257 = feedback #61() -> (w438:fxp<+/-,25,-2>)  [unwired: 1 in]
    n258 = feedback-in #61("frequency tracking k1.0") -> ()
    n259 = feedback #62() -> (w440:fxp<+/-,10,1>)  [unwired: 1 in]
    n260 = feedback-in #62("threshold precentile.0") -> ()
    n261 = feedback #63() -> (w441:i32)  [unwired: 1 in]
    n262 = feedback-in #63("preamble.0") -> ()
    n263 = Compound Arithmetic op=OR(w318, w455) -> (w385:bool)
    n264 = call "Detect Header.vi"("input data"=w310) -> ("header detected"=w328:bool, "timestamp"=w330:u64, "chdr_header"=w329:T2)  [unwired: 8 in]
    n265 = Compound Arithmetic op=AND(w328, w317) -> (w303:bool)
    n266 = feedback #64() -> (w358:bool)  [unwired: 1 in]
    n267 = call "PN Bit Stream with Preamble 8 BPC.vi"("preamble count"=w341, "ready for output"=w358, "on symbol count"=w349, "bit stream memory"=w334, "reset modulator"=w311, "start modulator"=w374, "preamble memory"=w335) -> ("output valid"=w363:bool, "data"=w362:fxp<+/-,16,1>[])  [unwired: 3 in]
    n268 = call "FIR Interpolate by 2 Polyphase 32 tap 4 SPC.vi"("filter coefficients even"=w361, "filter coefficients odd"=w360, "clock x2"=w333, "input valid"=w363, "data"=w362) -> ("output valid"=w365:bool, "data out"=w364:fxp<+/-,16,2>[])  [unwired: 5 in]
    n269 = call "Detect Packet Size Error.vi"("reset_pse"=w318, "end of frame"=w309, "input valid"=w317, "packet_header"=w303, "chdr_header"=w329) -> ("eof_misalignment_count"=w323:u64, "sequence errors"=w322:T14, "packet size errors"=w321:T15)  [unwired: 4 in]
    n270 = call "Add AWGN 8 SPC Imaginary Only.vi"("imaginary"=w364, "input valid"=w365, "power scaling"=w370, "reset"=w311, "seed"=w371, "scaling factor"=w372, "Output Type Selection"=w373) -> ("output with noise"=w356:u32[], "output valid"=w357:bool)  [unwired: 7 in]
    n271 = Bundle("packet size errors"=w321, "sequence errors"=w322, "eof_misalignment_count"=w323) -> (w325:T1)  [unwired: 1 in]
    n272 = call-poly <instrlib>:"Count Up.vi"("increment"=w303, "reset"=w318) -> ("count out"=w324:u64)  [unwired: 13 in]
    n273 = feedback #65() -> (→"last_header.0":T2)  [unwired: 1 in]
    n274 = feedback-in #65(w329, w303) -> ()
    n275 = feedback #66() -> (→"last_timestamp.0":u64)  [unwired: 1 in]
    n276 = feedback-in #66(w330, w303) -> ()
    n277 = feedback #67() -> (→"error detection.0":T1)  [unwired: 1 in]
    n278 = feedback-in #67(w325) -> ()
    n279 = feedback #68() -> (→"header count.0":u64)  [unwired: 1 in]
    n280 = feedback-in #68(w324) -> ()
    n281 = feedback #69() -> (w351:bool)  [unwired: 1 in]
    n282 = call "Pulse Output 8 SPC.vi"("Pulse Configuration"=w336, "reset"=w311, "enable"=w374, "ready for output"=w351, "input valid"=w357, "8 spc imaginary"=w356) -> ("Pulse Buffer Underflow"=w337:bool, "Ready for Input"=w338:bool, "output valid"=w381:bool, "IQ data out"=w308:u32[], "Number of Elements to Read"=w375:u32, "pulse buffer overflow"=w366:bool)
    n283 = feedback-in #64(w338) -> ()
    n284 = call-poly <instrlib>:"Number Array To Boolean Array.vi"("data in"=w308) -> ("data out"=w307:bool[])  [unwired: 14 in]
    n285 = feedback #70() -> (w378:T7)  [unwired: 1 in]
    n286 = feedback-in #70("header parameters.0") -> ()
    n287 = feedback #71() -> (w380:u16)  [unwired: 1 in]
    n288 = feedback-in #71("aurora frame length.0") -> ()
    n289 = Compound Arithmetic op=AND(w317, w304) -> (w302:bool)
    n290 = call-poly <instrlib>:"Boolean Array To Number Array.vi"("data in"=w310) -> ("data out"=w316:u32[])  [unwired: 14 in]
    n291 = feedback #72() -> (w383:bool)  [unwired: 1 in]
    n292 = call "256-bit CHDR Packetizer (Simple).vi"("ready for output"=w383, "reset"=w311, "aurora frame length"=w380, "input valid"=w381, "header parameters"=w378, "data"=w307) -> ("tlast"=w305:bool, "output valid"=w313:bool, "tkeep"=w306:bool[], "data out"=w314:bool[], "ready for input"=w382:bool)  [unwired: 1 in]
    n293 = feedback-in #69(w382) -> ()
    n294 = for {
      tunnel: w316 -> [w478] mode=indexing
      tunnel: [w477] -> w446 mode=indexing
      tunnel: [w476] -> w445 mode=indexing
      n295 = Split Number(x=w478) -> (hi(x)=w481:u16, lo(x)=w482:u16)
      n296 = Number To Boolean Array(number=w482) -> (Boolean array=w480:bool[])
      n297 = Number To Boolean Array(number=w481) -> (Boolean array=w479:bool[])
      n298 = Boolean Array To Number(Boolean array=w480) -> (number=w477:fxp<+/-,16,1>)
      n299 = Boolean Array To Number(Boolean array=w479) -> (number=w476:fxp<+/-,16,1>)
    }
    n300 = Compound Arithmetic op=AND(w302, invert w303) -> (w301:bool)
    n301 = call "FIR 32 tap 8 SPC.vi"("data in"=w446, "reset"=w385, "clock x2"=w384, "filter coefficients"=w447, "input valid"=w301) -> ("data out 16.1"=w402:fxp<+/-,16,1>[], "output valid"=w400:bool)  [unwired: 8 in, 1 out]
    n302 = call "FIR 32 tap 8 SPC.vi"("data in"=w445, "reset"=w385, "clock x2"=w384, "filter coefficients"=w447, "input valid"=w301) -> ("data out 16.1"=w401:fxp<+/-,16,1>[])  [unwired: 8 in, 2 out]
    n303 = Compound Arithmetic op=AND(invert w351, w381) -> (w347:bool)
    n304 = call-poly <vilib>:"Write Data Stream (Bit Array).vi"("endpoint"=w315, "reset"=w311, "end of frame"=w305, "input valid"=w313, "byte enable"=w306, "data"=w314) -> ("ready for input"=w312:bool)  [unwired: 5 in]
    n305 = feedback-in #72(w312) -> ()
    n306 = xnode ("FIFO Method Node")("Element"=w308, "Input Valid"=w381) -> ("Ready for Input"=w342:bool)  [unwired: 1 in, 1 out]
    n307 = call "AGC LPF 4spc.vi"("level threshold"=w389, "k 2"=w391, "level"=w390, "k 1"=w392, "reset"=w385, "input valid"=w400, "din img"=w401, "din real"=w402) -> ("AGC gain"=w387:fxp<+,19,3>, "current level"=w396:fxp<+,32,3>)  [unwired: 1 in, 1 out]
    n308 = call "AGC Apply Gain 8spc.vi"("AGC gain"=w387, "input valid"=w400, "din img"=w401, "din real"=w402) -> ("output valid"=w397:bool, "dout img"=w398:fxp<+/-,16,1>[], "dout real"=w399:fxp<+/-,16,1>[])  [unwired: 5 in]
    n309 = call "Burst Detection 8SPC.vi"("x real"=w399, "reset"=w385, "threshold precentile"=w440, "x img"=w398, "input valid"=w397, "preamble"=w441) -> ("Current Threshold"=w439:fxp<+/-,15,15>, "phase correction cos"=w430:fxp<+/-,16,2>, "phase correction sin"=w429:fxp<+/-,16,2>, "timing"=w436:fxp<+,13,0>, "img to interpolator"=w421:fxp<+/-,16,1>[], "real to interpolator"=w422:fxp<+/-,16,1>[], "preamble detected"=w419:bool)  [unwired: 2 in, 1 out]
    n310 = Build Array(w301) -> (w406:bool[])
    n311 = Compound Arithmetic op=AND(w419, w435) -> (w405:bool)
    n312 = Boolean Array To Number(Boolean array=w406) -> (number=w412:u8)
    n313 = Compound Arithmetic op=AND(invert w342, w381) -> (w343:bool)
    n314 = Compound Arithmetic op=AND(w405, w404) -> (w403:bool)
    n315 = call "Piecewise Parabolic Interpolation 8spc.vi"("x[n]"=w422, "u[k]"=w436, "reset"=w385, "preamble found"=w405, "input valid"=w397, "frame length"=w431) -> ("y[n]"=w427:fxp<+/-,16,2>[])  [unwired: 8 in, 1 out]
    n316 = call "Piecewise Parabolic Interpolation 8spc.vi"("x[n]"=w421, "u[k]"=w436, "reset"=w385, "preamble found"=w405, "input valid"=w397, "frame length"=w431) -> ("y[n]"=w426:fxp<+/-,16,2>[], "output valid"=w423:bool)  [unwired: 8 in]
    n317 = Initialize Array(u32 0 ("element"), 7 ("dimension size")) -> (w410:u32[])
    n318 = call <instrlib>:"Synchronous Latch.vi"("clear"=w352, "set"=w347) -> ("out"=w346:bool)  [unwired: 9 in]
    n319 = To Unsigned Long Integer(number=w412) -> (unsigned 32bit integer=w411:u32)
    n320 = call <instrlib>:"Synchronous Latch.vi"("clear"=w352, "set"=w343) -> ("out"=w344:bool)  [unwired: 9 in]
    n321 = call <instrlib>:"Detect Rising Edge.vi"("signal"=w403) -> ("edge detected"=w420:bool)  [unwired: 14 in]
    n322 = feedback #73() -> (→"pulse control overflow.0":bool)  [unwired: 1 in]
    n323 = feedback-in #73(w366) -> ()
    n324 = feedback #74() -> (→"pulse buffer underflow.0":bool)  [unwired: 1 in]
    n325 = feedback-in #74(w337) -> ()
    n326 = feedback #75() -> (→"output fifo elements.0":u32)  [unwired: 1 in]
    n327 = feedback-in #75(w375) -> ()
    n328 = feedback #76() -> (→"sink overflow.0":bool)  [unwired: 1 in]
    n329 = feedback-in #76(w346) -> ()
    n330 = feedback #77() -> (→"modulated data overflow.0":bool)  [unwired: 1 in]
    n331 = feedback-in #77(w344) -> ()
    n332 = call "Apply Phase Correction.vi"("phase correction cos"=w430, "phase correction sin"=w429, "input valid"=w423, "input img"=w426, "input real"=w427) -> ("output valid"=w442:bool, "output img"=w443:fxp<+/-,16,2>[], "output real"=w444:fxp<+/-,16,2>[])  [unwired: 4 in]
    n333 = Build Array (concatenate)(w316, w411, w410) -> (w407:u32[])
    n334 = call <instrlib>:"Synchronous Latch.vi"("clear"=w385, "set"=w420) -> ("out"=w413:bool)  [unwired: 9 in]
    n335 = call "BPSK Frequency Tracking 4SPC.vi"("I data in"=w444, "k1"=w438, "k2"=w437, "Q data in"=w443, "input valid"=w442, "reset"=w419) -> ("polar output"=w428:T16, "output valid"=w424:bool)  [unwired: 7 in, 1 out]
    n336 = for {
      tunnel: [w486] -> w425 mode=indexing
      tunnel: w428 -> [w485] mode=indexing
      n337 = Unbundle(w485) -> ("magnitude"=w484:fxp<+,16,2>, "phase"=w483:fxp<+/-,16,1>)  [unwired: 1 out]
      n338 = Number To Boolean Array(number=w484) -> (Boolean array=w490:bool[])
      n339 = Number To Boolean Array(number=w483) -> (Boolean array=w489:bool[])
      n340 = Boolean Array To Number(Boolean array=w490) -> (number=w488:u16)
      n341 = Boolean Array To Number(Boolean array=w489) -> (number=w487:u16)
      n342 = Join Numbers(hi=w488, lo=w487) -> ((hi.lo)=w486:u32)
    }
    n343 = call "Pulse BPSK Phase to Bits 4SPC.vi"("polar output"=w428, "input valid"=w424) -> ("bit"=w432:bool[], "output valid"=w434:bool)  [unwired: 12 in]
    n344 = Boolean Array To Number(Boolean array=w432) -> (number=w433:fxp<+,4,4>)
    n345 = xnode ("FIFO Method Node")("Element"=w432, "Input Valid"=w434) -> ("Ready for Input"=w459:bool)  [unwired: 1 in, 1 out]
    n346 = xnode ("FIFO Method Node")("Element"=w425, "Input Valid"=w424) -> ("Ready for Input"=w457:bool)  [unwired: 1 in, 1 out]
    n347 = xnode ("FIFO Write Using Handshaking")("Element"=w433, "Input Valid"=w434) -> ("Ready for Input"=w450:bool)  [unwired: 1 in, 1 out]
    n348 = xnode ("FIFO Method Node")("Element"=w407, "Input Valid"=w413) -> ("Ready for Input"=w418:bool)  [unwired: 1 in, 1 out]
    n349 = feedback #78() -> (w458:bool)  [unwired: 1 in]
    n350 = feedback-in #78(w459) -> ()
    n351 = feedback #79() -> (w456:bool)  [unwired: 1 in]
    n352 = feedback-in #79(w457) -> ()
    n353 = feedback #80() -> (w451:bool)  [unwired: 1 in]
    n354 = feedback-in #80(w450) -> ()
    n355 = feedback #81() -> (w414:bool)  [unwired: 1 in]
    n356 = feedback-in #81(w418) -> ()
    n357 = Compound Arithmetic op=AND(invert w458, w434) -> (w471:bool)
    n358 = Compound Arithmetic op=AND(invert w456, w424) -> (w468:bool)
    n359 = Compound Arithmetic op=AND(invert w451, w434) -> (w452:bool)
    n360 = Compound Arithmetic op=AND(invert w414, w413) -> (w415:bool)
    n361 = call <instrlib>:"Synchronous Latch.vi"("clear"=w385, "set"=w471) -> ("out"=w470:bool)  [unwired: 9 in]
    n362 = call <instrlib>:"Synchronous Latch.vi"("clear"=w385, "set"=w468) -> ("out"=w467:bool)  [unwired: 9 in]
    n363 = call <instrlib>:"Synchronous Latch.vi"("clear"=w385, "set"=w452) -> ("out"=w453:bool)  [unwired: 9 in]
    n364 = call <instrlib>:"Synchronous Latch.vi"("clear"=w385, "set"=w415) -> ("out"=w416:bool)  [unwired: 9 in]
    n365 = feedback #82() -> (→"current level.0":fxp<+,32,3>)  [unwired: 1 in]
    n366 = feedback-in #82(w396) -> ()
    n367 = feedback #83() -> (→"AGC gain.0":fxp<+,19,3>)  [unwired: 1 in]
    n368 = feedback-in #83(w387) -> ()
    n369 = feedback #84() -> (→"current threshold.0":fxp<+/-,15,15>)  [unwired: 1 in]
    n370 = feedback-in #84(w439) -> ()
    n371 = feedback #85() -> (→"demodulated bits overflow.0":bool)  [unwired: 1 in]
    n372 = feedback-in #85(w470) -> ()
    n373 = feedback #86() -> (→"constellation IQ overflow.0":bool)  [unwired: 1 in]
    n374 = feedback-in #86(w467) -> ()
    n375 = feedback #87() -> (→"demodulated bits to BER overflow.0":bool)  [unwired: 1 in]
    n376 = feedback-in #87(w453) -> ()
    n377 = feedback #88() -> (→"aurora.0":bool)  [unwired: 1 in]
    n378 = feedback-in #88(w416) -> ()
  }
  n379 = call <vilib>:"Read Register Bus Clock.vi"("endpoint collection"=w40) -> ("register bus clock"=w45:refnum<k21>)  [unwired: 10 in]
  n380 = call <vilib>:"Read FIFO Register Bus.vi"("endpoint collection"=w40) -> ("fifo register bus"=w46:refnum<class "niInstr FIFO Register Bus v1 FPGA.lvclass">)  [unwired: 10 in]
  n381 = call <vilib>:"Process.vi"("endpoint collection"=w40) -> ()  [unwired: 11 in]
  n382 = node-c288(w45) -> (w57:T10)
  n383 = node-c288(w23) -> (w25:T10)
  n384 = node-c288(w48) -> (w50:T10)
  n385 = timed-loop {
    timing: w57 -> [_]
    timing-out: [_] -> w56
    tunnel: w46 -> [w493]
    stop <- _ stop-if-true
    # "Instruction Framework Host Interface"
    n386 = call <instrlib>:"Host Interface.vi"("fifo register bus"=w493, "fifo reg bus ctrl 0"="fifo reg bus ctrl 0") -> ("fifo reg bus status 0"=→"fifo reg bus status 0":u32, "fifo reg bus data 0"=→"fifo reg bus data 0":u64)  [unwired: 12 in]
  }
  n387 = timed-loop {
    timing: w25 -> [_]
    timing-out: [_] -> w24
    tunnel: w17 -> [w502]
    stop <- _ stop-if-true
    # "Bit Error Rate Testing"
    n388 = xnode ("FIFO Read Using Handshaking")("Ready for Output"=TRUE) -> ("Element"=w501:fxp<+,4,4>, "Output Valid"=w500:bool)  [unwired: 1 in, 1 out]
    n389 = call "BER 4BPC.vi"("input valid"=w500, "input bits"=w501, "BER"=w502) -> ()  [unwired: 9 in]
  }
  n390 = timed-loop {
    timing: w50 -> [_]
    timing-out: [_] -> w49
    tunnel: w22 -> [w508]
    stop <- _ stop-if-true
    # "Bit Error Rate Testing"
    n391 = xnode ("FIFO Read Using Handshaking")("Ready for Output"=TRUE) -> ("Element"=w507:fxp<+,4,4>, "Output Valid"=w506:bool)  [unwired: 1 in, 1 out]
    n392 = call "BER 4BPC.vi"("input valid"=w506, "input bits"=w507, "BER"=w508) -> ()  [unwired: 9 in]
  }
  n393 = node-c288(w56) -> ()
  n394 = node-c288(w24) -> ()
  n395 = node-c288(w49) -> ()
  n396 = node-c288(w52) -> ()
  n397 = node-c288(w30) -> ()
  n398 = node-c288(w35) -> ()
  n399 = node-c288(w54) -> ()
